vi "Update Assert Data.vi"(8 "error in (no error)":errorcluster, 10 "Assert Data":T1, 11 "AssertEngine in":refnum<class "AssertEngine.lvclass">) -> (0 "error out":errorcluster, 3 "AssertEngine out":refnum<class "AssertEngine.lvclass">)   [LabVIEW 2016, in "AssertEngine.lvlib" / "AssertEngine.lvclass"]
uses:
  AssertEngine.lvclass
  Log Assert/Assert Data.ctl
  AssertEngine.lvclass/AssertEngine.ctl
  AssertEngine.lvlib
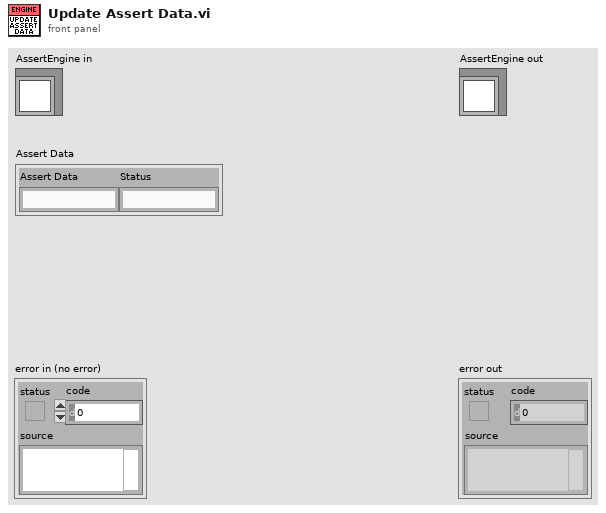
[diagram p1: front panel]
types:
  T1 = typedef "AssertEngine.lvlib/Assert Data.ctl" = cluster{"Assert Data":string, "Status":string}
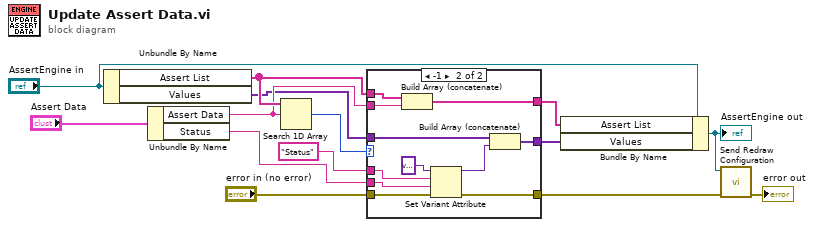
[diagram p0: block diagram]
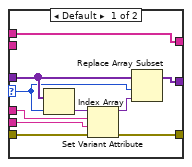
[diagram p2: hidden frame]
diagram:
  n1 = Unbundle By Name("AssertEngine in") -> ("Assert List"=w11:string[], "Values"=w9:variant[])
  n2 = Unbundle By Name("Assert Data") -> ("Assert Data"=w10:string, "Status"=w8:string)
  n3 = Search 1D Array(1D array=w11, element=w10) -> (index of element=w12:i32)  [unwired: 1 in]
  n4 = case shown="-1" w12 {
    selector: w12 -> [w16 _]
    tunnel: w11 -> [w24 w35]
    tunnel: w10 -> [_ w34]
    tunnel: [w24 w33] -> w4
    tunnel: w9 -> [w18 w29]
    tunnel: w8 -> [w19 w31]
    tunnel: "error in (no error)" -> [w22 w30]
    tunnel: "Status" ("name") -> [w20 w27]
    tunnel: [w21 w26] -> w5
    tunnel: [w15 w25] -> w3
    frame Default {
      n5 = Index Array(array=w18, index=w16) -> (element=w23:variant)
      n6 = Set Variant Attribute(Variant=w23, name=w20, value=w19, error in=w22) -> (Variant out=w17:variant, error out=w21:errorcluster)  [unwired: 1 out]
      n7 = Replace Array Subset(array=w18, new element=w17, index=w16) -> (w15:variant[])
    }
    frame -1 {
      n8 = Build Array (concatenate)(w35, w34) -> (w33:string[])
      n9 = Set Variant Attribute(Variant=variant, name=w27, value=w31, error in=w30) -> (Variant out=w28:variant, error out=w26:errorcluster)  [unwired: 1 out]
      n10 = Build Array (concatenate)(w29, w28) -> (w25:variant[])
    }
  }
  n11 = Bundle By Name(cluster="AssertEngine in", "Assert List"=w4, "Values"=w3) -> (w1:refnum<class "AssertEngine.lvclass">)
  "AssertEngine out" <- w1
  n12 = call "Send Redraw Configuration.vi"("error in (no error)"=w5, "AssertEngine in"=w1) -> ("error out"=→"error out":errorcluster)  [unwired: 9 in]
